vi "Change State.vi"(8 "error in (no error)":errorcluster, 10 "New State in":refnum<class "State Actor.lvclass">, 11 "State in":refnum<class "State Actor.lvclass">) -> (0 "error out":errorcluster, 3 "State out":refnum<class "State Actor.lvclass">)   [LabVIEW 2012, in "State Actor.lvclass"]
doc: "This method defines state transitions; use it to construct the specific state transitions of your State Pattern Actor. \n\nThe method takes the current state and the next state as inputs. It invokes Exit.vi on the current state. It then invokes Substitute Actor.vi to transfer data from the current state to the next state. Finally, it invokes Entry.vi on the new state, and returns that state as the current state."
uses:
  State Actor.lvclass
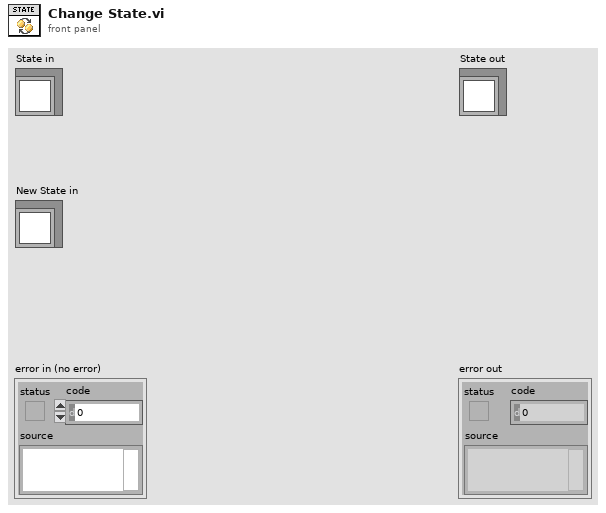
[diagram p1: front panel]
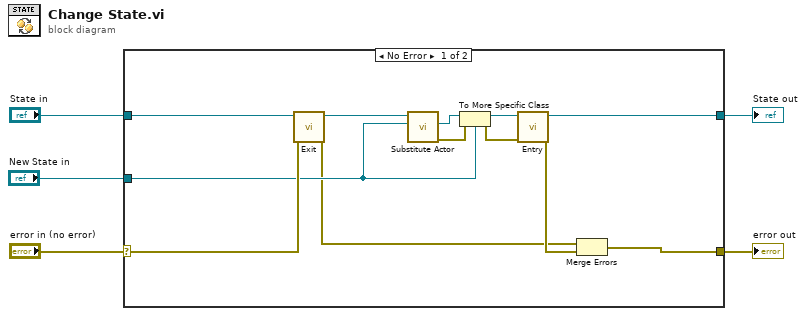
[diagram p0: block diagram]
diagram:
  n1 = case shown="No Error" "error in (no error)" {
    selector: "error in (no error)" -> [w16 w19]
    tunnel: [w7 w19] -> w3
    tunnel: [w15 w18] -> w4
    tunnel: "State in" -> [w17 w18]
    tunnel: "New State in" -> [w11 _]
    frame No Error {
      n2 = call-dynamic "Exit.vi"("error in (no error)"=w16, "Old State"=w17) -> ("error out"=w6:errorcluster, "New State"=w13:refnum<class "State Actor.lvclass">)  [unwired: 8 in]
      n3 = call-dynamic "Substitute Actor.vi"("Substitute Actor in"=w11, "Current Actor"=w13) -> ("error out"=w9:errorcluster, "Substitute Actor out"=w10:refnum<class "Actor.lvclass">)  [unwired: 8 in]
      n4 = To More Specific Class(target class=w11, reference=w10, error in=w9) -> (specific class reference=w12:refnum<class "State Actor.lvclass">, error out=w8:errorcluster)
      n5 = call-dynamic "Entry.vi"("error in (no error)"=w8, "New State"=w12) -> ("error out"=w14:errorcluster, "State out"=w15:refnum<class "State Actor.lvclass">)  [unwired: 8 in]
      n6 = Merge Errors(w6, w14) -> (w7:errorcluster)
    }
    frame Error {
    }
  }
  "error out" <- w3
  "State out" <- w4
